vi "Multi Axis Query.vi"(0 "System no.":i32, 5 "Command":string, 7 "Axis":string[](array[string]), 9 "All axes?":bool, 11 "error in (no error)":errorcluster) -> (4 "Answer":string, 15 "error out":errorcluster)   [LabVIEW 2020]
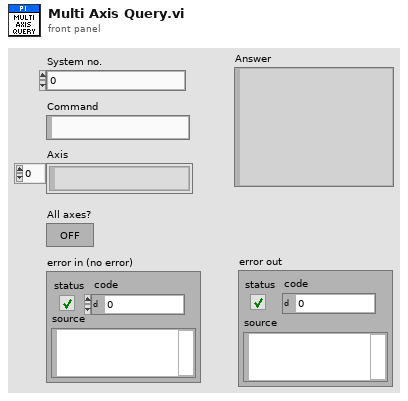
[diagram p1: front panel]
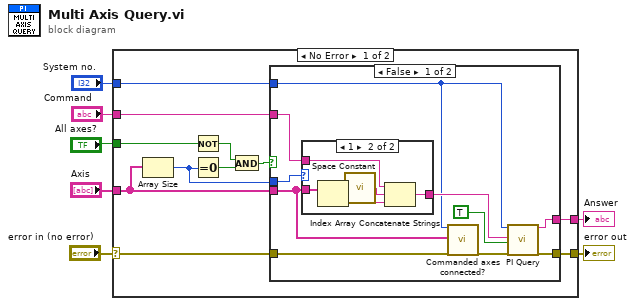
[diagram p0: block diagram]
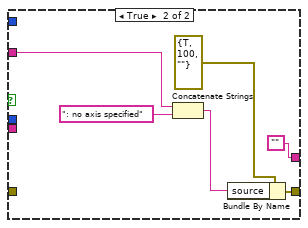
[diagram p3: hidden frame]
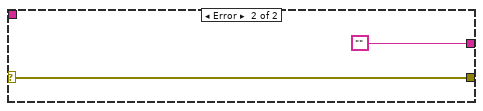
[diagram p4: hidden frame]
diagram:
  n1 = case shown="No Error" "error in (no error)" {
    selector: "error in (no error)" -> [w10 w42]
    tunnel: [w18 "" ("String read")] -> w7
    tunnel: "Axis" -> [w17 _]
    tunnel: [w16 w42] -> w5
    tunnel: "Command" -> [w15 _]
    tunnel: "All axes?" -> [w9 _]
    tunnel: "System no." -> [w8 _]
    frame No Error {
      n2 = Array Size(array=w17) -> (size(s)=w14:i32)
      n3 = Not(x=w9) -> (.not. x?=w11:bool)
      n4 = Equal To 0?(x=w14) -> (x = 0?=w13:bool)
      n5 = And(x=w11, y=w13) -> (x .and. y?=w12:bool)
      n6 = case shown="False" w12 {
        tunnel: w8 -> [w23 _]
        tunnel: w17 -> [w22 _]
        tunnel: w10 -> [w25 _]
        tunnel: [w19 w39] -> w16
        tunnel: w14 -> [w24 _]
        tunnel: w15 -> [w21 w36]
        tunnel: [w20 "" ("String read")] -> w18
        frame False {
          n7 = case shown="1" w24 {
            tunnel: [w29 w34] -> w27
            tunnel: w22 -> [_ w33]
            tunnel: w21 -> [w29 w32]
            frame 0, Default {
            }
            frame 1 {
              n8 = Index Array(array=w33) -> (element=w31:string)  [unwired: 1 in]
              n9 = call <vilib>:"Space Constant.vi"() -> ("String"=w30:string)
              n10 = Concatenate Strings(w32, w30, w31) -> (w34:string)
            }
          }
          n11 = call "Commanded axes connected?.vi"("System no."=w23, "Commanded axes"=w22, "error in"=w25) -> ("error out"=w26:errorcluster)  [unwired: 1 in, 15 out]
          n12 = call "PI Query.vi"("System no."=w23, "String to send"=w27, "Attach termination char.?"=TRUE ("Attach Linefeed?"), "error in"=w26) -> ("String read"=w20:string, "error out"=w19:errorcluster)  [unwired: 3 in, 11 out]
        }
        frame True {
          n13 = Concatenate Strings(w36, ": no axis specified" ("source")) -> (w38:string)
          n14 = Bundle By Name(cluster=errorcluster {"status"=TRUE, "code"=100, "source"=""} ("error out"), "source"=w38) -> (w39:errorcluster)
        }
      }
    }
    frame Error {
    }
  }
  "Answer" <- w7
  "error out" <- w5
